vi "icon_url.get.vi"(8 "error in (no error)":errorcluster, 11 "workspace in":refnum<class "workspace.lvclass">) -> (0 "error out":errorcluster, 2 "icon url":string, 3 "workspace out":refnum<class "workspace.lvclass">)   [LabVIEW 2020, in "nominal types.lvlib" / "workspace.lvclass"]
uses:
  workspace.lvclass
  workspace.lvclass/workspace.ctl
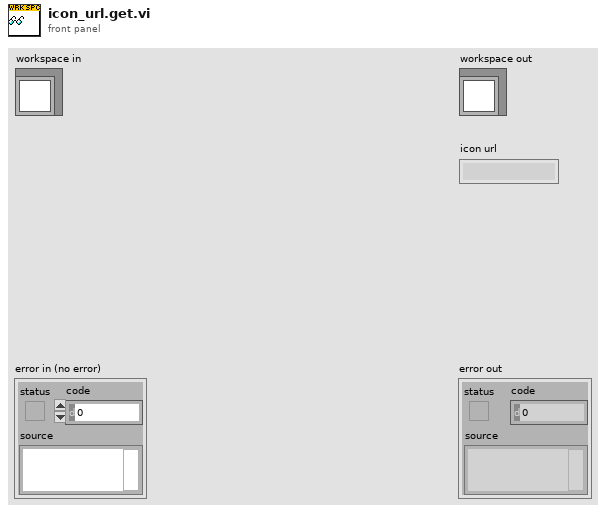
[diagram p1: front panel]
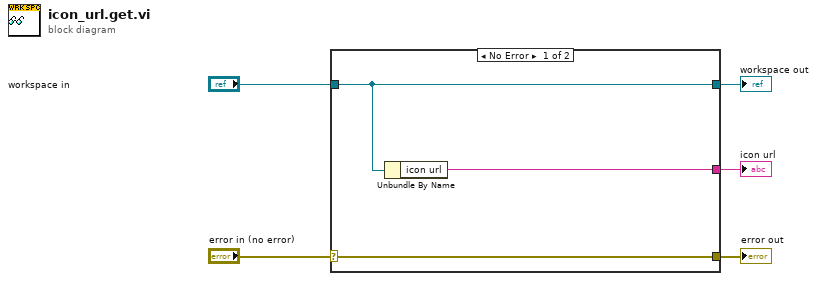
[diagram p0: block diagram]
diagram:
  n1 = case shown="No Error" "error in (no error)" {
    selector: "error in (no error)" -> [w8 w9]
    tunnel: [w8 w9] -> w4
    tunnel: [w7 w10] -> w2
    tunnel: "workspace in" -> [w7 w10]
    tunnel: [w6 _] -> w1
    frame No Error {
      n2 = Unbundle By Name(w7) -> ("icon url"=w6:string)
    }
    frame Error {
    }
  }
  "error out" <- w4
  "workspace out" <- w2
  "icon url" <- w1
